vi "Add State.vi"(8 "error in (no error)":errorcluster, 9 "Name":string, 10 "Cal Folder":path, 11 "Tosca in":refnum<class "Parameters.lvclass">) -> (0 "error out":errorcluster, 3 "Tosca out":refnum<class "Parameters.lvclass">)   [LabVIEW 2015, in "Parameters.lvclass"]
uses:
  Parameters.lvclass
  Parameters.lvclass/Parameters.ctl
  State/State.lvclass
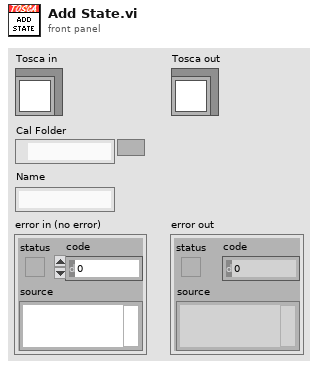
[diagram p1: front panel]
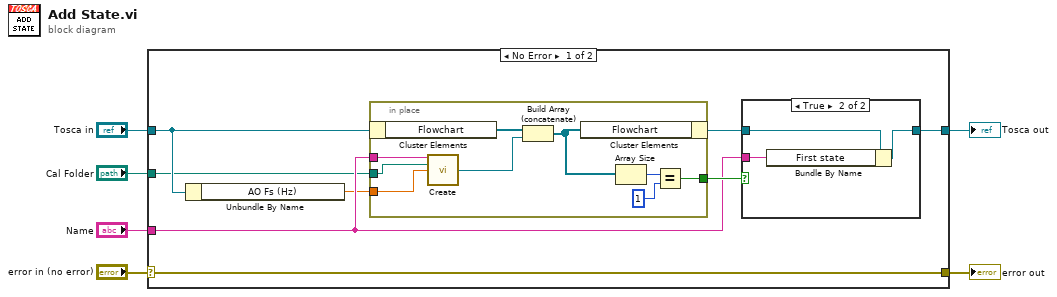
[diagram p0: block diagram]
diagram:
  n1 = case shown="No Error" "error in (no error)" {
    selector: "error in (no error)" -> [w14 w29]
    tunnel: [w14 w29] -> w5
    tunnel: [w10 w28] -> w3
    tunnel: "Tosca in" -> [w9 w28]
    tunnel: "Name" -> [w11 _]
    tunnel: "Cal Folder" -> [w7 _]
    frame No Error {
      n2 = Unbundle By Name(w9) -> ("AO Fs (Hz)"=w8:dbl)
      n3 = in-place {
        in-place-border: w11 -> [w21]
        in-place-border: [w22] -> w13
        in-place-border: w8 -> [w20]
        in-place-border: w7 -> [w19]
        n4 = in-place-cluster #1(w9) -> ("Flowchart"=w27:refnum<class "State.lvclass">[])
        n5 = call "Create.vi"("Name"=w21, "Cal Folder"=w19, "Fs (Hz)"=w20) -> ("State"=w26:refnum<class "State.lvclass">)  [unwired: 12 in]
        n6 = Build Array (concatenate)(w27, w26) -> (w25:refnum<class "State.lvclass">[])
        n7 = in-place-cluster #1("Flowchart"=w25) -> (w12:refnum<class "Parameters.lvclass">)
        n8 = Array Size(array=w25) -> (size(s)=w24:i32)
        n9 = Equal?(x=w24, y=1) -> (x = y?=w22:bool)
      }
      n10 = case shown="True" w13 {
        tunnel: w12 -> [w15 w18]
        tunnel: [w15 w17] -> w10
        tunnel: w11 -> [_ w16]
        frame False {
        }
        frame True {
          n11 = Bundle By Name(cluster=w18, "First state"=w16) -> (w17:refnum<class "Parameters.lvclass">)
        }
      }
    }
    frame Error {
    }
  }
  "error out" <- w5
  "Tosca out" <- w3
